vi "create_cache_if_nonexistent.vi"(8 "error in (no error)":errorcluster, 10 "cache file":path, 11 "exists":bool) -> (0 "error out":errorcluster, 3 "cache file path":path)   [LabVIEW 2016]
uses:
  <userlib>/_OpenG.lib/file/file.llb/Strip Path - Traditional__ogtk.vi
  <userlib>/_OpenG.lib/file/file.llb/Build Path - Traditional__ogtk.vi
panel:
  out "created folders":bool
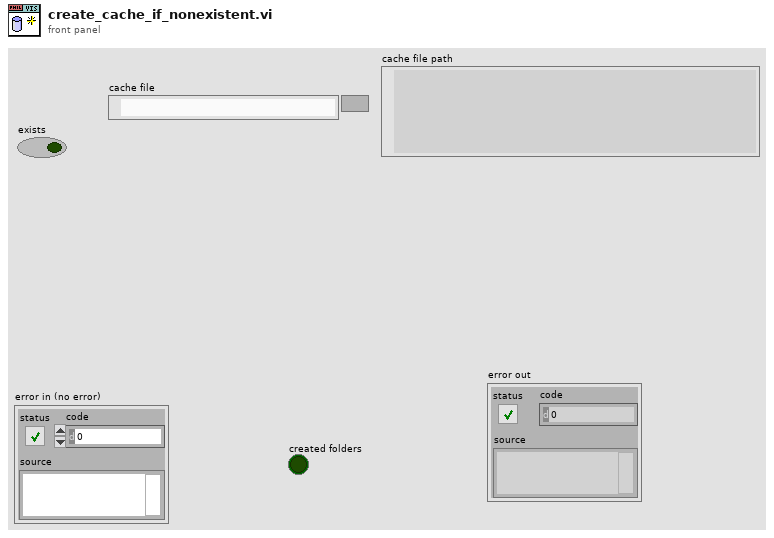
[diagram p1: front panel]
types:
  T1 = enum16{"open", "replace", "create", "open or create", "replace or create", "replace or create with confirmation"}
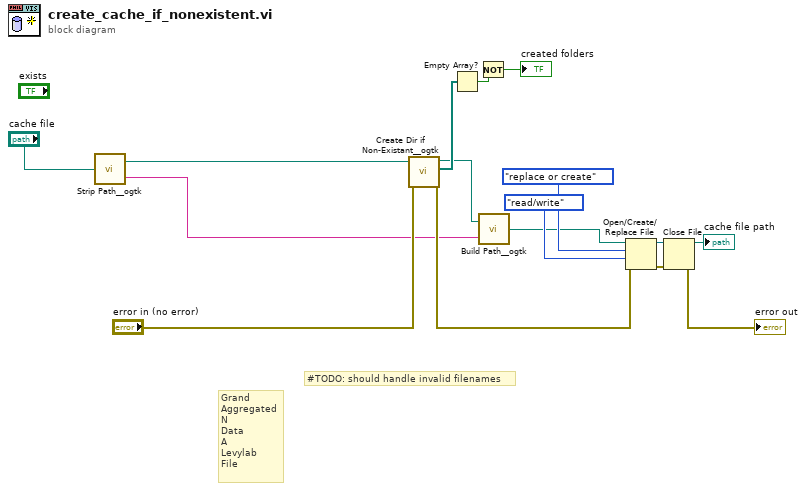
[diagram p0: block diagram]
diagram:
  # "Grand\nAggregated\nN\nData\nA\nLevylab\nFile"
  # "#TODO: should handle invalid filenames"
  n1 = call-poly <userlib>:"Strip Path__ogtk.vi"("path"="cache file") -> ("stripped path"=w4:path, "name"=w3:string)
  n2 = call <userlib>:"Create Dir if Non-Existant__ogtk.vi"("error in (no error)"="error in (no error)", "Directory Path"=w4) -> ("error out"=w8:errorcluster, "Created Directories"=w15:path[], "dup Directory Path"=w12:path)  [unwired: 7 in]
  n3 = Empty Array?(array=w15) -> (empty?=w14:bool)
  n4 = Not(x=w14) -> (.not. x?=→"created folders":bool)
  n5 = call-poly <userlib>:"Build Path__ogtk.vi"("name or relative path"=w3, "base path"=w12) -> ("appended path"=w9:path)
  n6 = Open/Create/Replace File(file path (use dialog)=w9, error in=w8, operation (0:open)=T1."replace or create", access (0:read/write)=enum16{"read/write", "read-only", "write-only"}."read/write") -> (refnum out=w1:refnum<file>, error out=w2:errorcluster)  [unwired: 2 in, 1 out]
  n7 = Close File(refnum=w1, error in=w2) -> (path=→"cache file path":path, error out=→"error out":errorcluster)
